vi "manual ramping query.vi"(8 "error in (no error)":errorcluster, 11 "VISA session":refnum<visa-resource-name>) -> (0 "error out":errorcluster, 2 "Ramping":bool, 3 "dup VISA session":refnum<visa-resource-name>)   [LabVIEW 2023]
panel:
  out "Setpoint":dbl[unit]
  out "Field Reading 2":dbl
  out "Field Reading":dbl
  out "slope":bool
  out "field":bool
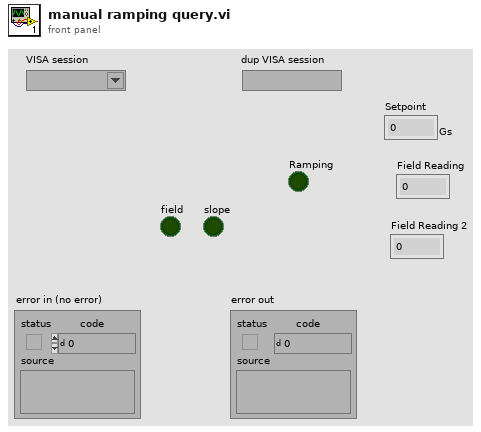
[diagram p1: front panel]
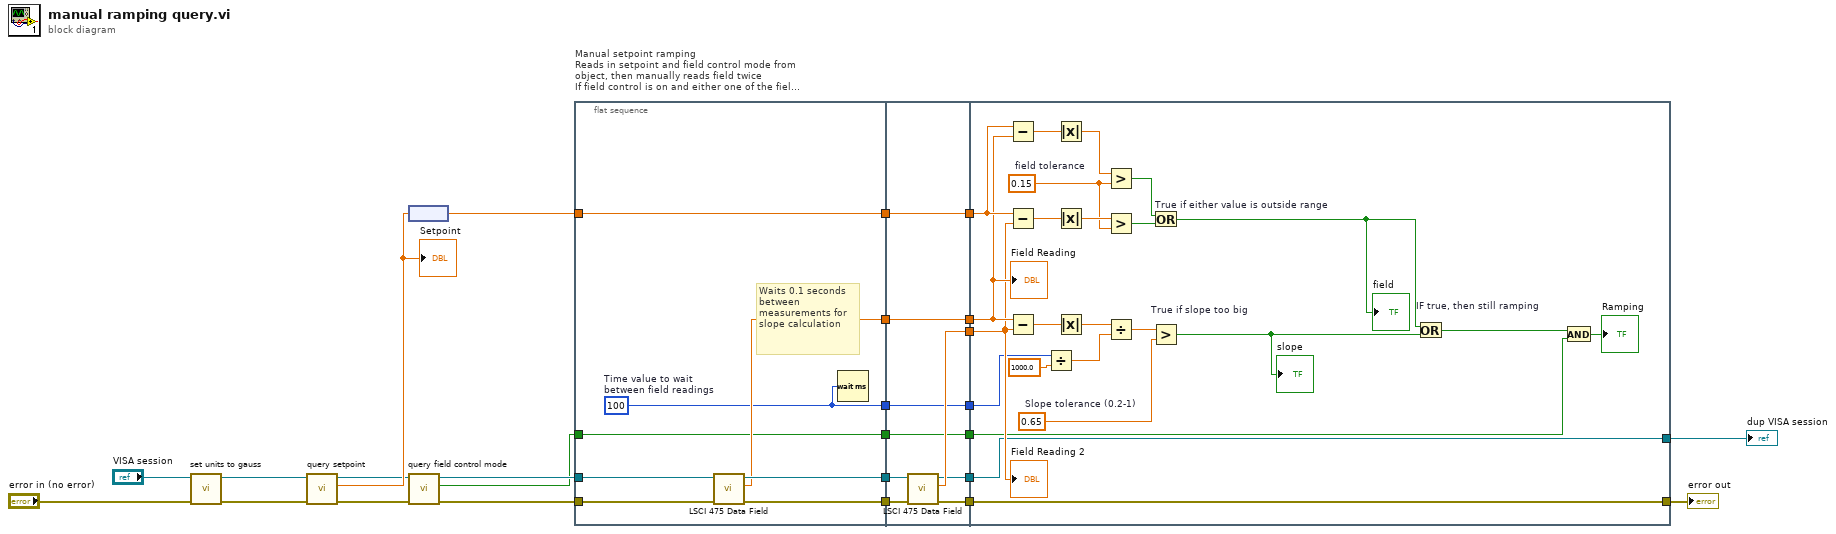
[diagram p0: block diagram]
diagram:
  n1 = call "set units to gauss.vi"("VISA session"="VISA session", "error in (no error)"="error in (no error)") -> ("dup VISA session"=w8:refnum<visa-resource-name>, "error out"=w7:errorcluster)  [unwired: 7 in]
  n2 = call "query setpoint.vi"("error in (no error)"=w7, "VISA session"=w8) -> ("error out"=w3:errorcluster, "Setpoint"=w6:dbl[unit], "dup VISA session"=w5:refnum<visa-resource-name>)  [unwired: 7 in]
  "Setpoint" <- w6
  n3 = node(w6) -> (w13:dbl)
  n4 = call "query field control mode.vi"("error in (no error)"=w3, "VISA session"=w5) -> ("error out"=w2:errorcluster, "Controlling field?"=w1:bool, "dup VISA session"=w4:refnum<visa-resource-name>)  [unwired: 7 in]
  n5 = flat-sequence "Manual setpoint ramping\nReads in setpoint and field control mode from object, then manually reads field twice\nIf field control is on and either one of the field measurements or slope is outside of the acceptable range, then ramping is true\nIf field control is off, or it's on and all of the measurements are within acceptable range, then ramping is false" {
    tunnel: w4 -> [w32]
    tunnel: w2 -> [w34]
    tunnel: [w33] -> w26
    tunnel: [w31] -> w25
    tunnel: [w30] -> w24
    tunnel: w13 -> [w30]
    tunnel: [w29] -> w23
    tunnel: [w28] -> w22
    tunnel: w1 -> [w28]
    tunnel: [w27] -> w9
    tunnel: w26 -> [w43]
    tunnel: w25 -> [w42]
    tunnel: [w41] -> w21
    tunnel: w24 -> [w41]
    tunnel: [w40] -> w20
    tunnel: w23 -> [w40]
    tunnel: [w39] -> w19
    tunnel: [w38] -> w18
    tunnel: w22 -> [w38]
    tunnel: [w37] -> w17
    tunnel: [w36] -> w16
    tunnel: [w35] -> w10
    tunnel: w9 -> [w35]
    tunnel: w21 -> [w58]
    tunnel: w20 -> [w57]
    tunnel: w19 -> [w56]
    tunnel: w18 -> [w45]
    tunnel: w17 -> [w55]
    tunnel: w16 -> [w54]
    tunnel: [w55] -> w15
    tunnel: [w54] -> w14
    tunnel: w10 -> [w50]
    frame #0 {
      w27 = u32 100  # Time value to wait between field readings
      # "Waits 0.1 seconds between measurements for slope calculation"
      n6 = call "LSCI 475 Data Field.vi"("error in (no error)"=w34, "VISA session"=w32) -> ("error out"=w33:errorcluster, "Field Reading"=w29:dbl, "dup VISA session"=w31:refnum<visa-resource-name>)  [unwired: 7 in]
      n7 = Wait (ms)(milliseconds to wait=w27) -> ()  [unwired: 1 out]
    }
    frame #1 {
      n8 = call "LSCI 475 Data Field.vi"("error in (no error)"=w43, "VISA session"=w42) -> ("error out"=w36:errorcluster, "Field Reading"=w39:dbl, "dup VISA session"=w37:refnum<visa-resource-name>)  [unwired: 7 in]
    }
    frame #2 {
      w59 = 0.65  # Slope tolerance (0.2-1)
      w63 = 0.15  # field tolerance
      n9 = Subtract(x=w58, y=w57) -> (x-y=w67:dbl)
      n10 = Subtract(x=w58, y=w56) -> (x-y=w66:dbl)
      n11 = Subtract(x=w57, y=w56) -> (x-y=w48:dbl)
      n12 = Divide(x=w50, y=1000.0) -> (x/y=w49:dbl)
      n13 = Absolute Value(x=w67) -> (abs(x)=w65:dbl)
      n14 = Absolute Value(x=w66) -> (abs(x)=w64:dbl)
      n15 = Absolute Value(x=w48) -> (abs(x)=w47:dbl)
      n16 = Greater?(x=w65, y=w63) -> (0:w62:bool)
      n17 = Greater?(x=w64, y=w63) -> (0:w61:bool)
      n18 = Divide(x=w47, y=w49) -> (x/y=w60:dbl)
      n19 = Or "True if either value is outside range"(x=w62, y=w61) -> (x .or. y?=w53:bool)
      "field" <- w53
      n20 = Greater? "True if slope too big"(x=w60, y=w59) -> (0:w52:bool)
      "slope" <- w52
      n21 = Or "IF true, then still ramping"(x=w53, y=w52) -> (x .or. y?=w46:bool)
      n22 = And(x=w46, y=w45) -> (x .and. y?=→"Ramping":bool)
      "Field Reading" <- w57
      "Field Reading 2" <- w56
    }
  }
  "dup VISA session" <- w15
  "error out" <- w14
